vi "FormatObstacles.vi"(7 "map in":i32[][](array[numeric]), 9 "Intensity of object":i32, 10 "Obstacles":T1) -> (0 "map out":i32[][](array[numeric]))   [LabVIEW 2011]
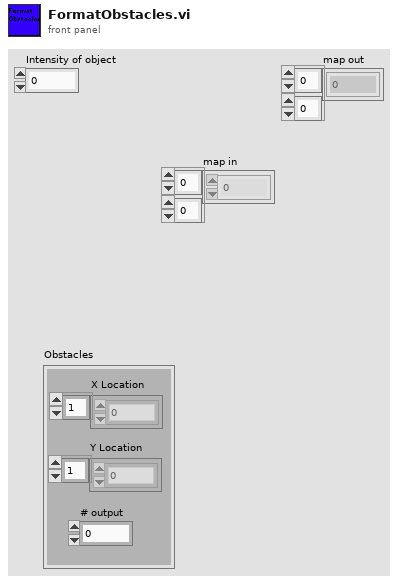
[diagram p1: front panel]
types:
  T1 = cluster{"X Location":dbl[], "Y Location":dbl[], "# output":i32}
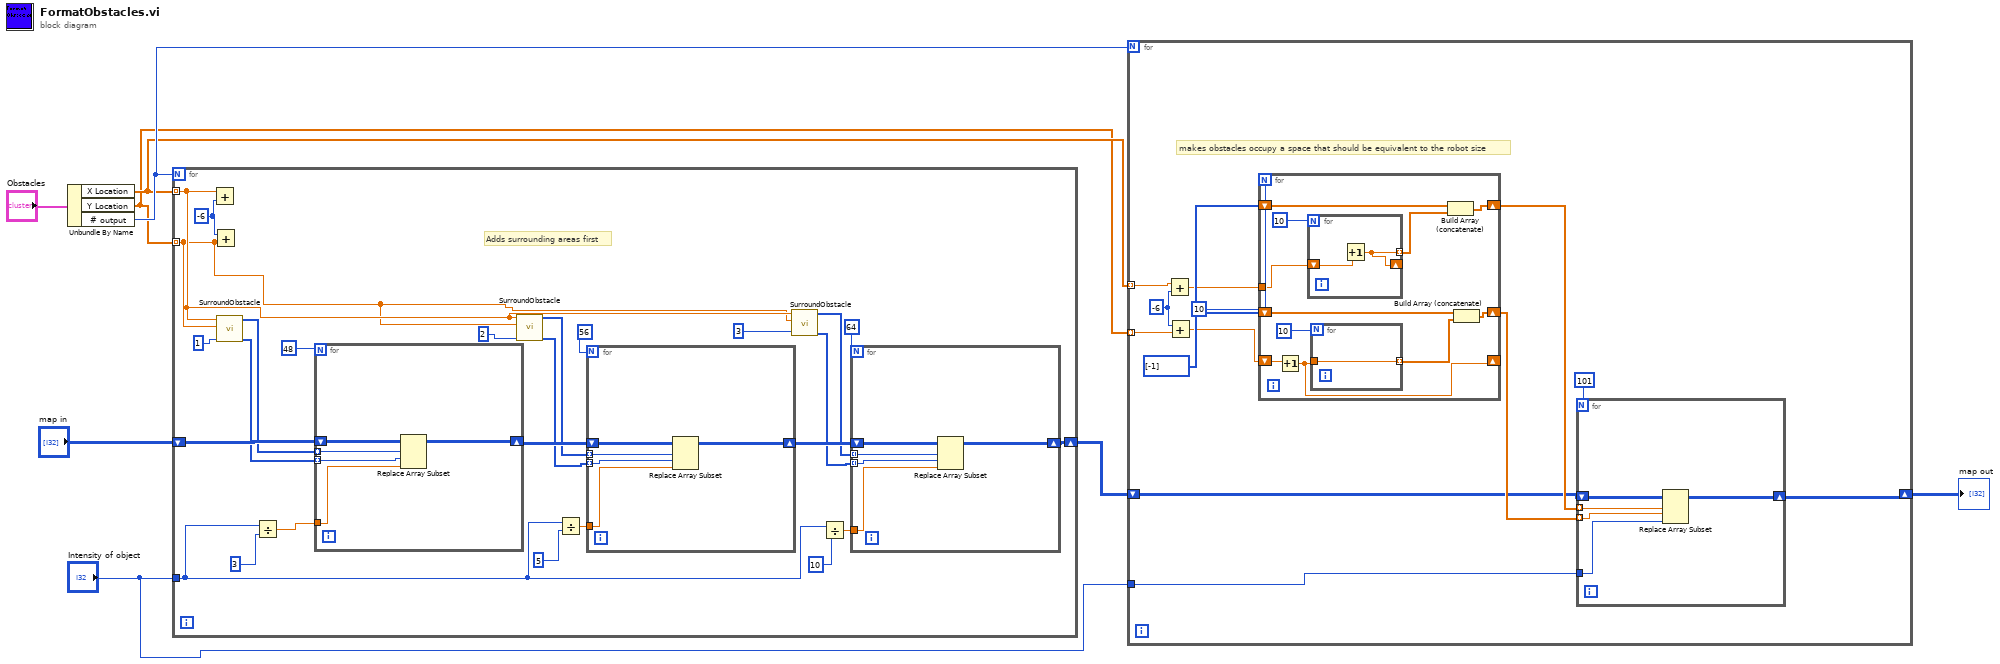
[diagram p0: block diagram]
diagram:
  n1 = Unbundle By Name("Obstacles") -> ("X Location"=w5:dbl[], "Y Location"=w4:dbl[], "# output"=w6:i32)
  n2 = for {
    N: w6 -> [_]
    tunnel: w5 -> [w14] mode=indexing
    tunnel: w4 -> [w13] mode=indexing
    shift-right: [w9] -> w7
    shift-left: "map in" -> [w31]
    tunnel: "Intensity of object" -> [w23]
    w34 = -6
    # "Adds surrounding areas first"
    n3 = Add(x=w14, y=w34) -> ()  [unwired: 1 out]
    n4 = Add(x=w34, y=w13) -> ()  [unwired: 1 out]
    n5 = call "SurroundObstacle.vi"("outside layer +1"=1, "y"=w13, "x"=w14) -> ("y array"=w19:i32[], "x array"=w20:i32[])  [unwired: 7 in]
    n6 = Divide(x=w23, y=3) -> (x/y=w27:dbl)
    n7 = for {
      N: 48 -> [_]
      shift-right: [w39] -> w32
      shift-left: w31 -> [w38]
      tunnel: w27 -> [w35]
      tunnel: w20 -> [w37] mode=indexing
      tunnel: w19 -> [w36] mode=indexing
      n8 = Replace Array Subset(array=w38, new element=w35, index (row)=w37, index (col)=w36) -> (w39:i32[][])
    }
    n9 = call "SurroundObstacle.vi"("outside layer +1"=2, "y"=w13, "x"=w14) -> ("y array"=w17:i32[], "x array"=w18:i32[])  [unwired: 7 in]
    n10 = Divide(x=w23, y=5) -> (x/y=w21:dbl)
    n11 = for {
      N: 56 -> [_]
      shift-right: [w44] -> w33
      shift-left: w32 -> [w43]
      tunnel: w21 -> [w40]
      tunnel: w18 -> [w42] mode=indexing
      tunnel: w17 -> [w41] mode=indexing
      n12 = Replace Array Subset(array=w43, new element=w40, index (row)=w42, index (col)=w41) -> (w44:i32[][])
    }
    n13 = call "SurroundObstacle.vi"("outside layer +1"=3, "y"=w13, "x"=w14) -> ("y array"=w15:i32[], "x array"=w16:i32[])  [unwired: 7 in]
    n14 = Divide(x=w23, y=10) -> (x/y=w22:dbl)
    n15 = for {
      N: 64 -> [_]
      shift-right: [w49] -> w9
      shift-left: w33 -> [w48]
      tunnel: w22 -> [w45]
      tunnel: w16 -> [w47] mode=indexing
      tunnel: w15 -> [w46] mode=indexing
      n16 = Replace Array Subset(array=w48, new element=w45, index (row)=w47, index (col)=w46) -> (w49:i32[][])
    }
  }
  n17 = for {
    N: w6 -> [_]
    shift-right: [w56] -> w2
    shift-left: w7 -> [w55]
    tunnel: w5 -> [w54] mode=indexing
    tunnel: w4 -> [w53] mode=indexing
    tunnel: "Intensity of object" -> [w52]
    w62 = -6
    w60 = i32[] [-1]
    # "makes obstacles occupy a space that should be equivalent to the robot size"
    n18 = Add(x=w54, y=w62) -> (x+y=w50:dbl)
    n19 = Add(x=w62, y=w53) -> (x+y=w51:dbl)
    n20 = for {
      N: 10 -> [_]
      shift-right: [w71] -> w61
      shift-left: w60 -> [w70]
      shift-right: [w68] -> w59
      shift-left: w60 -> [w67]
      shift-right: [w64] -> _
      shift-left: w51 -> [w65]
      tunnel: w50 -> [w63]
      n21 = Increment(x=w65) -> (x+1=w64:dbl)
      n22 = for {
        N: 10 -> [_]
        tunnel: [w75] -> w69 mode=indexing
        shift-right: [w75] -> _
        shift-left: w63 -> [w76]
        n23 = Increment(x=w76) -> (x+1=w75:dbl)
      }
      n24 = for {
        N: 10 -> [_]
        tunnel: w64 -> [w74]
        tunnel: [w74] -> w66 mode=indexing
      }
      n25 = Build Array (concatenate)(w67, w69) -> (w68:dbl[])
      n26 = Build Array (concatenate)(w70, w66) -> (w71:dbl[])
    }
    n27 = for {
      N: 101 -> [_]
      shift-right: [w81] -> w56
      shift-left: w55 -> [w78]
      tunnel: w59 -> [w79] mode=indexing
      tunnel: w61 -> [w80] mode=indexing
      tunnel: w52 -> [w77]
      n28 = Replace Array Subset(array=w78, new element=w77, index (row)=w79, index (col)=w80) -> (w81:i32[][])
    }
  }
  "map out" <- w2
